vi "Init control.vi"(7 "ctl in":refnum<class "ctl.lvclass">, 8 "error in":errorcluster, 11 "Template Name":string) -> (0 "error out":errorcluster, 3 "ctl out":refnum<class "ctl.lvclass">)   [LabVIEW 2012, in "ctl.lvclass"]
uses:
  ctl.lvclass
  ctl.lvclass/ctl.ctl
  <userlib>/_OpenG.lib/file/file.llb/Strip Path Extension - 1D Array of Strings__ogtk.vi
  _ResManager_v86/IDCloneResMgr.lvlib
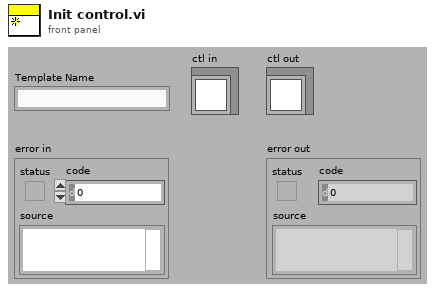
[diagram p1: front panel]
types:
  T1 = typedef "IDCloneResMgr.lvlib/ID_Resource info.ctl" = cluster{"type":u32, "id":i32, "name":string, "binary data":string}
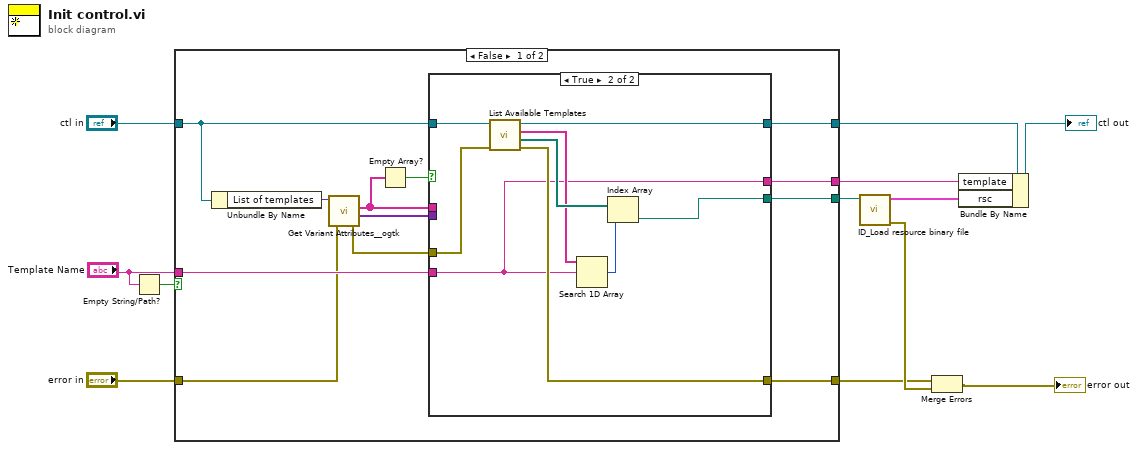
[diagram p0: block diagram]
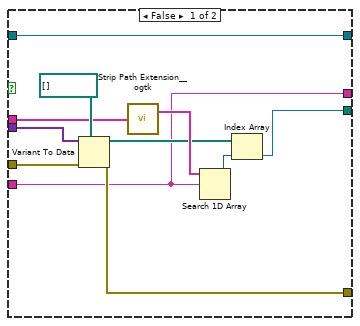
[diagram p2: hidden frame]
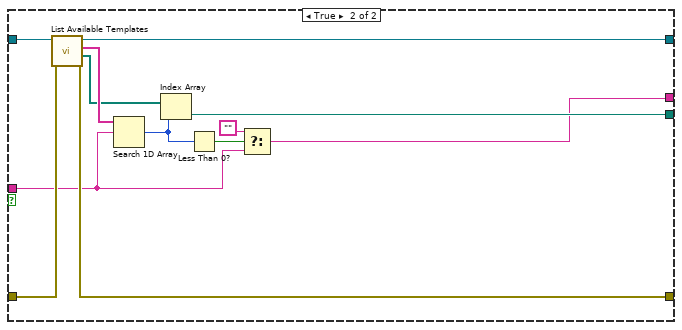
[diagram p3: hidden frame]
diagram:
  n1 = Empty String/Path?(string/path="Template Name") -> (empty?=w4:bool)
  n2 = case shown="False" w4 {
    tunnel: "ctl in" -> [w15 w56]
    tunnel: [w14 w55] -> w7
    tunnel: "Template Name" -> [w21 w47]
    tunnel: [w22 w52] -> w6
    tunnel: "error in" -> [w19 w51]
    tunnel: [w18 w50] -> w2
    tunnel: [w13 w45] -> w1
    frame False {
      n3 = Unbundle By Name(w15) -> ("List of templates"=w23:variant)
      n4 = call <userlib>:"Get Variant Attributes__ogtk.vi"("error in"=w19, "Variant"=w23) -> ("error out"=w20:errorcluster, "value(s)"=w24:variant[], "names"=w17:string[])  [unwired: 2 in, 1 out]
      n5 = Empty Array?(array=w17) -> (empty?=w16:bool)
      n6 = case shown="True" w16 {
        tunnel: w24 -> [w35 _]
        tunnel: [w30 w36] -> w22
        tunnel: w21 -> [w26 w37]
        tunnel: w20 -> [w29 w42]
        tunnel: [w28 w41] -> w18
        tunnel: w17 -> [w27 _]
        tunnel: w15 -> [w25 w44]
        tunnel: [w25 w43] -> w14
        tunnel: [w26 w37] -> w13
        frame False {
          n7 = Variant To Data(error in=w29, type=path[] [], Variant=w35) -> (data=w32:path[], error out=w28:errorcluster)
          n8 = call-poly <userlib>:"Strip Path Extension__ogtk.vi"("paths"=w27) -> ("roots"=w33:string[])  [unwired: 1 out]
          n9 = Search 1D Array(1D array=w33, element=w26) -> (index of element=w31:i32)  [unwired: 1 in]
          n10 = Index Array(array=w32, index=w31) -> (element=w30:path)
        }
        frame True {
          n11 = call "List Available Templates.vi"("error in (no error)"=w42, "ctl in"=w44) -> ("error out"=w41:errorcluster, "Templates Paths"=w39:path[], "Templates Available"=w38:string[], "ctl out"=w43:refnum<class "ctl.lvclass">)  [unwired: 6 in]
          n12 = Search 1D Array(1D array=w38, element=w37) -> (index of element=w40:i32)  [unwired: 1 in]
          n13 = Index Array(array=w39, index=w40) -> (element=w36:path)
        }
      }
    }
    frame True {
      n14 = call "List Available Templates.vi"("error in (no error)"=w51, "ctl in"=w56) -> ("error out"=w50:errorcluster, "Templates Paths"=w53:path[], "Templates Available"=w54:string[], "ctl out"=w55:refnum<class "ctl.lvclass">)  [unwired: 6 in]
      n15 = Search 1D Array(1D array=w54, element=w47) -> (index of element=w49:i32)  [unwired: 1 in]
      n16 = Index Array(array=w53, index=w49) -> (element=w52:path)
      n17 = Less Than 0?(x=w49) -> (x < 0?=w48:bool)
      n18 = Select(t="", s=w48, f=w47) -> (s? t:f=w45:string)
    }
  }
  n19 = call "ID_Load resource binary file.vi"("resource binary file"=w6) -> ("error out"=w10:errorcluster, "resources"=w9:T1[])  [unwired: 9 out]
  n20 = Merge Errors(w2, w10) -> (→"error out":errorcluster)
  n21 = Bundle By Name(cluster=w7, "template"=w1, "rsc"=w9) -> (→"ctl out":refnum<class "ctl.lvclass">)
